vi "纳清氨氮_所有参数读取.vi"(8 "error in (no error)":errorcluster caption="错误输入（无错误）", 11 "MB session in":refnum<class "MB_Master.lvclass">) -> (0 "error out":errorcluster caption="错误输出", 2 "输出值":T1 {"校准参数类型" items=["参数1校准"=1, "参数2校准"=2, "参数3校准"=3, "参数4校准"=4]; "波特率" items=["4800", "9600", "19200", "38400", "57600", "115200"]}, 3 "MB session out":refnum<class "MB_Master.lvclass">)   [LabVIEW 2016, in "斯坦道多参数.lvlib"]
uses:
  <vilib>/Plasmionique/MB Master/MB_Master/MB_Master.lvclass
  <vilib>/Plasmionique/MB Master/MB Master.lvlib
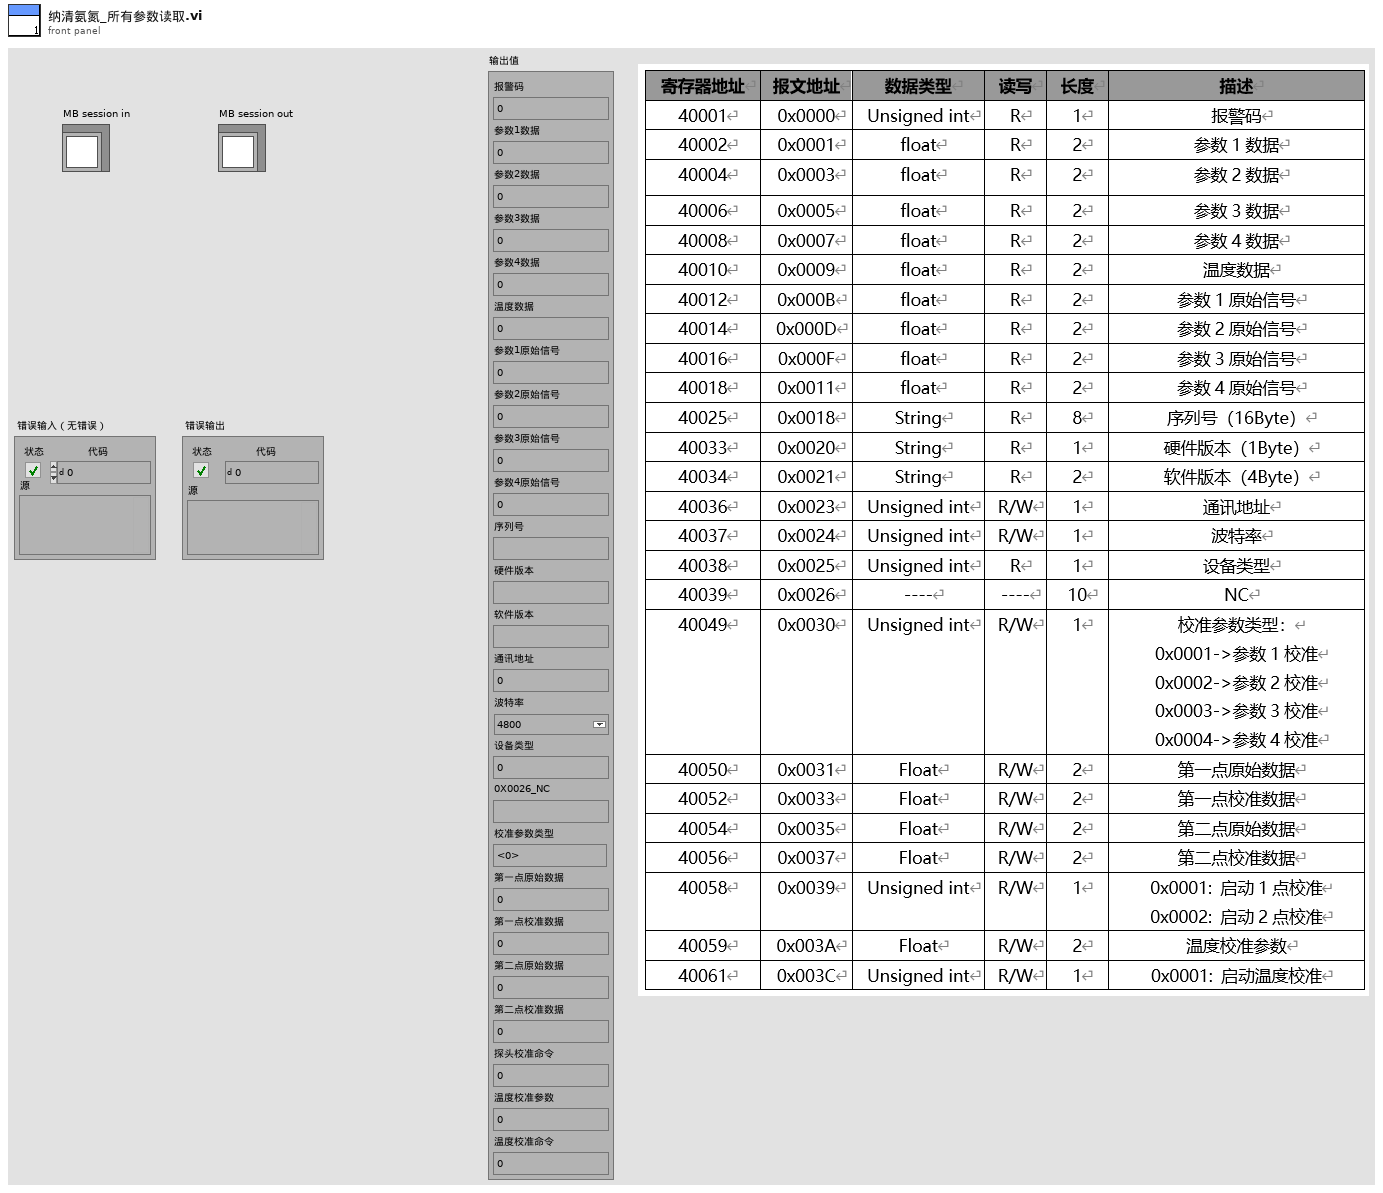
[diagram p1: front panel]
types:
  T1 = cluster{"报警码":u16, "参数1数据":sgl, "参数2数据":sgl, "参数3数据":sgl, "参数4数据":sgl, "温度数据":sgl, "参数1原始信号":sgl, "参数2原始信号":sgl, "参数3原始信号":sgl, "参数4原始信号":sgl, "序列号":string, "硬件版本":string, "软件版本":string, "通讯地址":u16, "波特率":u16, "设备类型":u16, "0X0026_NC":string, "校准参数类型":u16, "第一点原始数据":sgl, "第一点校准数据":sgl, "第二点原始数据":sgl, "第二点校准数据":sgl, "探头校准命令":u16, "温度校准参数":sgl, "温度校准命令":u16}
  T2 = cluster{"pH":u32, "DO":u32, "Cond":u32, "Turb":u32, "叶绿素a":u32, "藻密度":u32, "ORP":u32, "COD":u32, "氯化物":u32, "氨氮":u32, "水中油":u32}
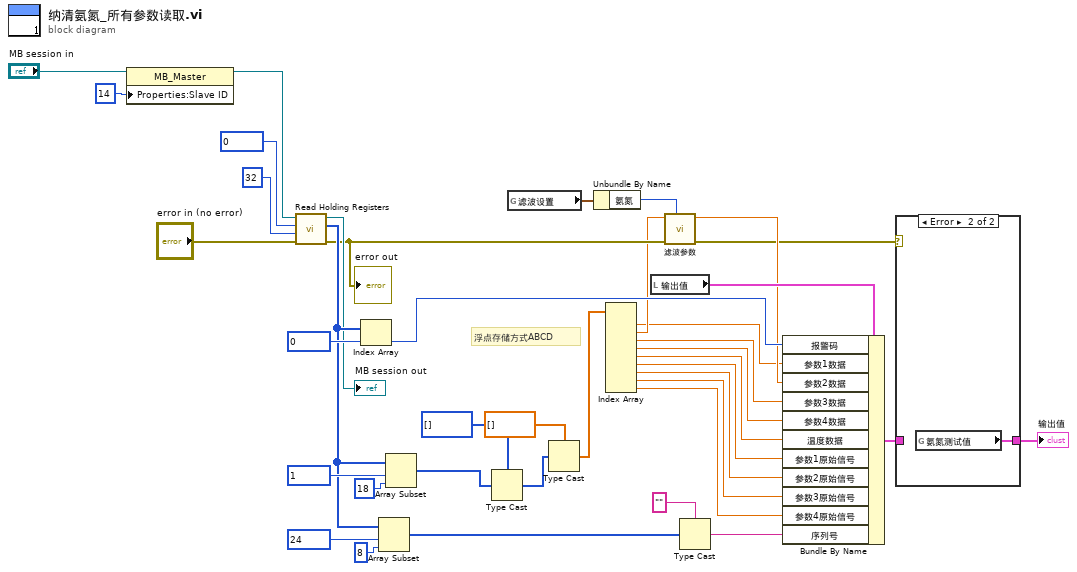
[diagram p0: block diagram]
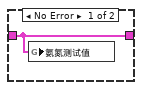
[diagram p2: hidden frame]
diagram:
  # "浮点存储方式ABCD"
  n1 = property class="MB_Master"(reference="MB session in", "Properties:Slave ID"=u8 14 ("Slave ID")) -> (reference out=w29:refnum<class "MB_Master.lvclass">)  [unwired: 1 in, 1 out]
  n2 = call <vilib>:"Read Holding Registers.vi"("error in (no error)"="error in (no error)", "quantity"=u16 32, "starting address"=u16 0, "MB session in"=w29) -> ("error out"=w14:errorcluster, "Registers"=w22:u16[], "MB session out"=→"MB session out":refnum<class "MB_Master.lvclass">)  [unwired: 5 in]
  "error out" <- w14
  n3 = Index Array(array=w22, index=u16 0 ("starting address")) -> (element=w37:u16)
  n4 = Array Subset(array=w22, index=u16 24 ("starting address"), length=8 ("长度")) -> (w24:u16[])
  n5 = Array Subset(array=w22, index=u16 1 ("starting address"), length=18 ("长度")) -> (w33:u16[])
  n6 = Type Cast(type=u32[] [] ("数组 2"), x=w33) -> (*(type *) &x=w21:u32[])
  n7 = global read "断电保存变量.vi" "滤波设置"() -> (w16:T2)
  n8 = Type Cast(type=sgl[] [] ("数组 2"), x=w21) -> (*(type *) &x=w32:sgl[])
  n9 = Unbundle By Name(w16) -> ("氨氮"=w15:u32)
  n10 = Index Array(array=w32) -> (element #1=w2:sgl, element #2=w4:sgl, element #3=w18:sgl, element #4=w17:sgl, element #5=w9:sgl, element #6=w8:sgl, element #7=w7:sgl, element #8=w6:sgl, element #9=w5:sgl)  [unwired: 9 in]
  n11 = local read "输出值"() -> (w12:T1)
  n12 = call "滤波参数.vi"("滤波次数"=w15, "error in (no error)"=w14, "x"=w4) -> ("error out"=w1:errorcluster, "mode"=w3:dbl)  [unwired: 7 in]
  n13 = Type Cast(type="" ("类型"), x=w24) -> (*(type *) &x=w10:string)
  n14 = Bundle By Name(cluster=w12, "报警码"=w37, "参数1数据"=w2, "参数2数据"=w3, "参数3数据"=w18, "参数4数据"=w17, "温度数据"=w9, "参数1原始信号"=w8, "参数2原始信号"=w7, "参数3原始信号"=w6, "参数4原始信号"=w5, "序列号"=w10) -> (w11:T1)
  n15 = case shown="Error" w1 {
    tunnel: [w40 w41] -> w13
    tunnel: w11 -> [w40 _]
    frame No Error {
      n16 = global write "纳清过程全局变量.vi" "氨氮测试值"(w40) -> ()
    }
    frame Error {
      n17 = global read "纳清过程全局变量.vi" "氨氮测试值"() -> (w41:T1)
    }
  }
  "输出值" <- w13
